vi "PhotonVision_ReadTargetData.vi"() -> ()   [LabVIEW 2019]
uses:
  <vilib>/Rock Robotics/WPI/ThirdParty/PhotonVisionLib/PhotonVisionLib.lvlib
  <vilib>/Rock Robotics/WPI/ThirdParty/JAS_Junk/TrajLib/Trajectory_Library.lvlib
  <vilib>/Rock Robotics/Network Tables/NT Write Number.vi
  <vilib>/Rock Robotics/Network Tables/NT Write Boolean.vi
  <vilib>/Rock Robotics/Network Tables/NT Write String.vi
  <vilib>/Rock Robotics/Network Tables/NT Write Integer.vi
  <vilib>/Rock Robotics/Network Tables/NT Write Numeric Array.vi
  <vilib>/Analysis/Matrix/NI_Matrix.lvlib
  <vilib>/Analysis/Matrix/Numeric/Conversions/Matrix To Array - RM.vi
  <vilib>/Rock Robotics/Network Tables/NT Read Boolean.vi
  <vilib>/Rock Robotics/Network Tables/NT Read Integer.vi
  <vilib>/Rock Robotics/WPI/ThirdParty/PhotonVisionLib/TypeDef/TargetCornerType.ctl
  <vilib>/Rock Robotics/WPI/ThirdParty/JAS_Junk/TrajLib/TypeDef/TRANSLATION3D.ctl
  <vilib>/Rock Robotics/WPI/ThirdParty/JAS_Junk/TrajLib/TypeDef/QUATERNION.ctl
  <vilib>/Rock Robotics/WPI/ThirdParty/JAS_Junk/TrajLib/TypeDef/ROTATION3D.ctl
  <vilib>/Rock Robotics/WPI/ThirdParty/JAS_Junk/TrajLib/TypeDef/TRANSFORM3D.ctl
  <vilib>/Rock Robotics/WPI/ThirdParty/PhotonVisionLib/TypeDef/PhotonTrackedTargetType.ctl
  <vilib>/Rock Robotics/WPI/ThirdParty/PhotonVisionLib/TypeDef/PhotonPipelineResultType.ctl
  <vilib>/Rock Robotics/WPI/ThirdParty/PhotonVisionLib/TypeDef/PhotonPNPResultType.ctl
  <vilib>/Rock Robotics/WPI/ThirdParty/PhotonVisionLib/TypeDef/PhotonMultiTargetPNPResultType.ctl
  <vilib>/Rock Robotics/WPI/ThirdParty/VisionLEDModeType.ctl
  <vilib>/Analysis/Matrix/Datatypes/RealMatrix.ctl
panel:
  in  "LEDMode Request":T1
  out "PipelineIndexReq":i64
  in  "PipelineIndex\nRequest":i32
  out "OutputSnapCmd":i64
  out "InputSnapCmd":i64
  in  "OutputSnapshot":bool
  in  "Input Snapshot":bool
  out "DriverModeRequest":bool
  in  "DriverMode":bool
  out "Dist Coeffs":T2
  out "CameraMatrix":T2
  out "IsConnected 2":bool
  out "PipelineIndex":i32
  out "DriverMode":bool
  out "Version":string
  out "LEDMode":T1
  out "size(s)":i32
  out "unsigned byte array":u8[](array[numeric])
  out "error out":errorcluster
  out "New Data":bool
  out "IsConnected":bool
  out "Has Targets":bool
  in  "CameraName":string="HD_Pro_Webcam_C920"
  out "CtrlLibDistToBestTarg\nMeters":dbl
  out "Loop Count":i32
  out "SpecificPhotonTrackedTarget":T3={"Yaw"=0.0, "Pitch"=0.0, "Area"=0.0, "Skew"=0.0, "MinAreaRectCorners"=[], "BestCameraToTarget"={"TRANSLATION3D"={"X"=0.0, "Y"=0.0, "Z"=0.0}, "ROTATION3D"={"Q_quaternion"={"R"=1.0, "V"=[0.0, 0.0, 0.0]}}, "XF"=FALSE}, "FiiducialId"=0, "AltCameraToTarget"={"TRANSLATION3D"={"X"=0.0, "Y"=0.0, "Z"=0.0}, "ROTATION3D"={"Q_quaternion"={"R"=0.0, "V"=[0.0, 0.0, 0.0]}}, "XF"=FALSE}, "PoseAmbiguity"=0.0, "DetectedCorners"=[]} {"AltCameraToTarget"."TRANSLATION3D"."Z" format="%14.3f"; "AltCameraToTarget"."TRANSLATION3D"."Y" format="%14.3f"; "AltCameraToTarget"."TRANSLATION3D"."X" format="%14.3f"; "BestCameraToTarget"."TRANSLATION3D"."Z" format="%14.3f"; "BestCameraToTarget"."TRANSLATION3D"."Y" format="%14.3f"; "BestCameraToTarget"."TRANSLATION3D"."X" format="%14.3f"}
  out "PipelineResult":T9={"TargetCount"=0, "Latency_MilliSec"=0.0, "Targets"=[], "TimeStampSec"=0.0, "PhotonMultiTargetPNPResult"={"PhotonPNPResult"={"IsPresent"=FALSE, "bestReprojErr"=0.0, "altReprojErr"=0.0, "ambiguity"=0.0, "Best"={"TRANSLATION3D"={"X"=0.0, "Y"=0.0, "Z"=0.0}, "ROTATION3D"={"Q_quaternion"={"R"=1.0, "V"=[0.0, 0.0, 0.0]}}, "XF"=FALSE}, "Alt"={"TRANSLATION3D"={"X"=0.0, "Y"=0.0, "Z"=0.0}, "ROTATION3D"={"Q_quaternion"={"R"=1.0, "V"=[0.0, 0.0, 0.0]}}, "XF"=FALSE}}, "FiducialIDsUsed"=[]}} {"PhotonMultiTargetPNPResult"."PhotonPNPResult"."Alt"."TRANSLATION3D"."Z" format="%14.3f"; "PhotonMultiTargetPNPResult"."PhotonPNPResult"."Alt"."TRANSLATION3D"."Y" format="%14.3f"; "PhotonMultiTargetPNPResult"."PhotonPNPResult"."Alt"."TRANSLATION3D"."X" format="%14.3f"; "PhotonMultiTargetPNPResult"."PhotonPNPResult"."Best"."TRANSLATION3D"."Z" format="%14.3f"; "PhotonMultiTargetPNPResult"."PhotonPNPResult"."Best"."TRANSLATION3D"."Y" format="%14.3f"; "PhotonMultiTargetPNPResult"."PhotonPNPResult"."Best"."TRANSLATION3D"."X" format="%14.3f"; "Targets"."AltCameraToTarget"."TRANSLATION3D"."Z" format="%14.3f"; "Targets"."AltCameraToTarget"."TRANSLATION3D"."Y" format="%14.3f"; "Targets"."AltCameraToTarget"."TRANSLATION3D"."X" format="%14.3f"; "Targets"."BestCameraToTarget"."TRANSLATION3D"."Z" format="%14.3f"; "Targets"."BestCameraToTarget"."TRANSLATION3D"."Y" format="%14.3f"; "Targets"."BestCameraToTarget"."TRANSLATION3D"."X" format="%14.3f"}
  out "SpecificTargetFound":bool
  out "TagTarget Index":i32
  in  "Fiiducial ID\n(April Tag Number)":i32
  out "BestTargetFound":bool
  out "BestYaw":dbl
  out "DistanceToBestTarget \nMeters":dbl
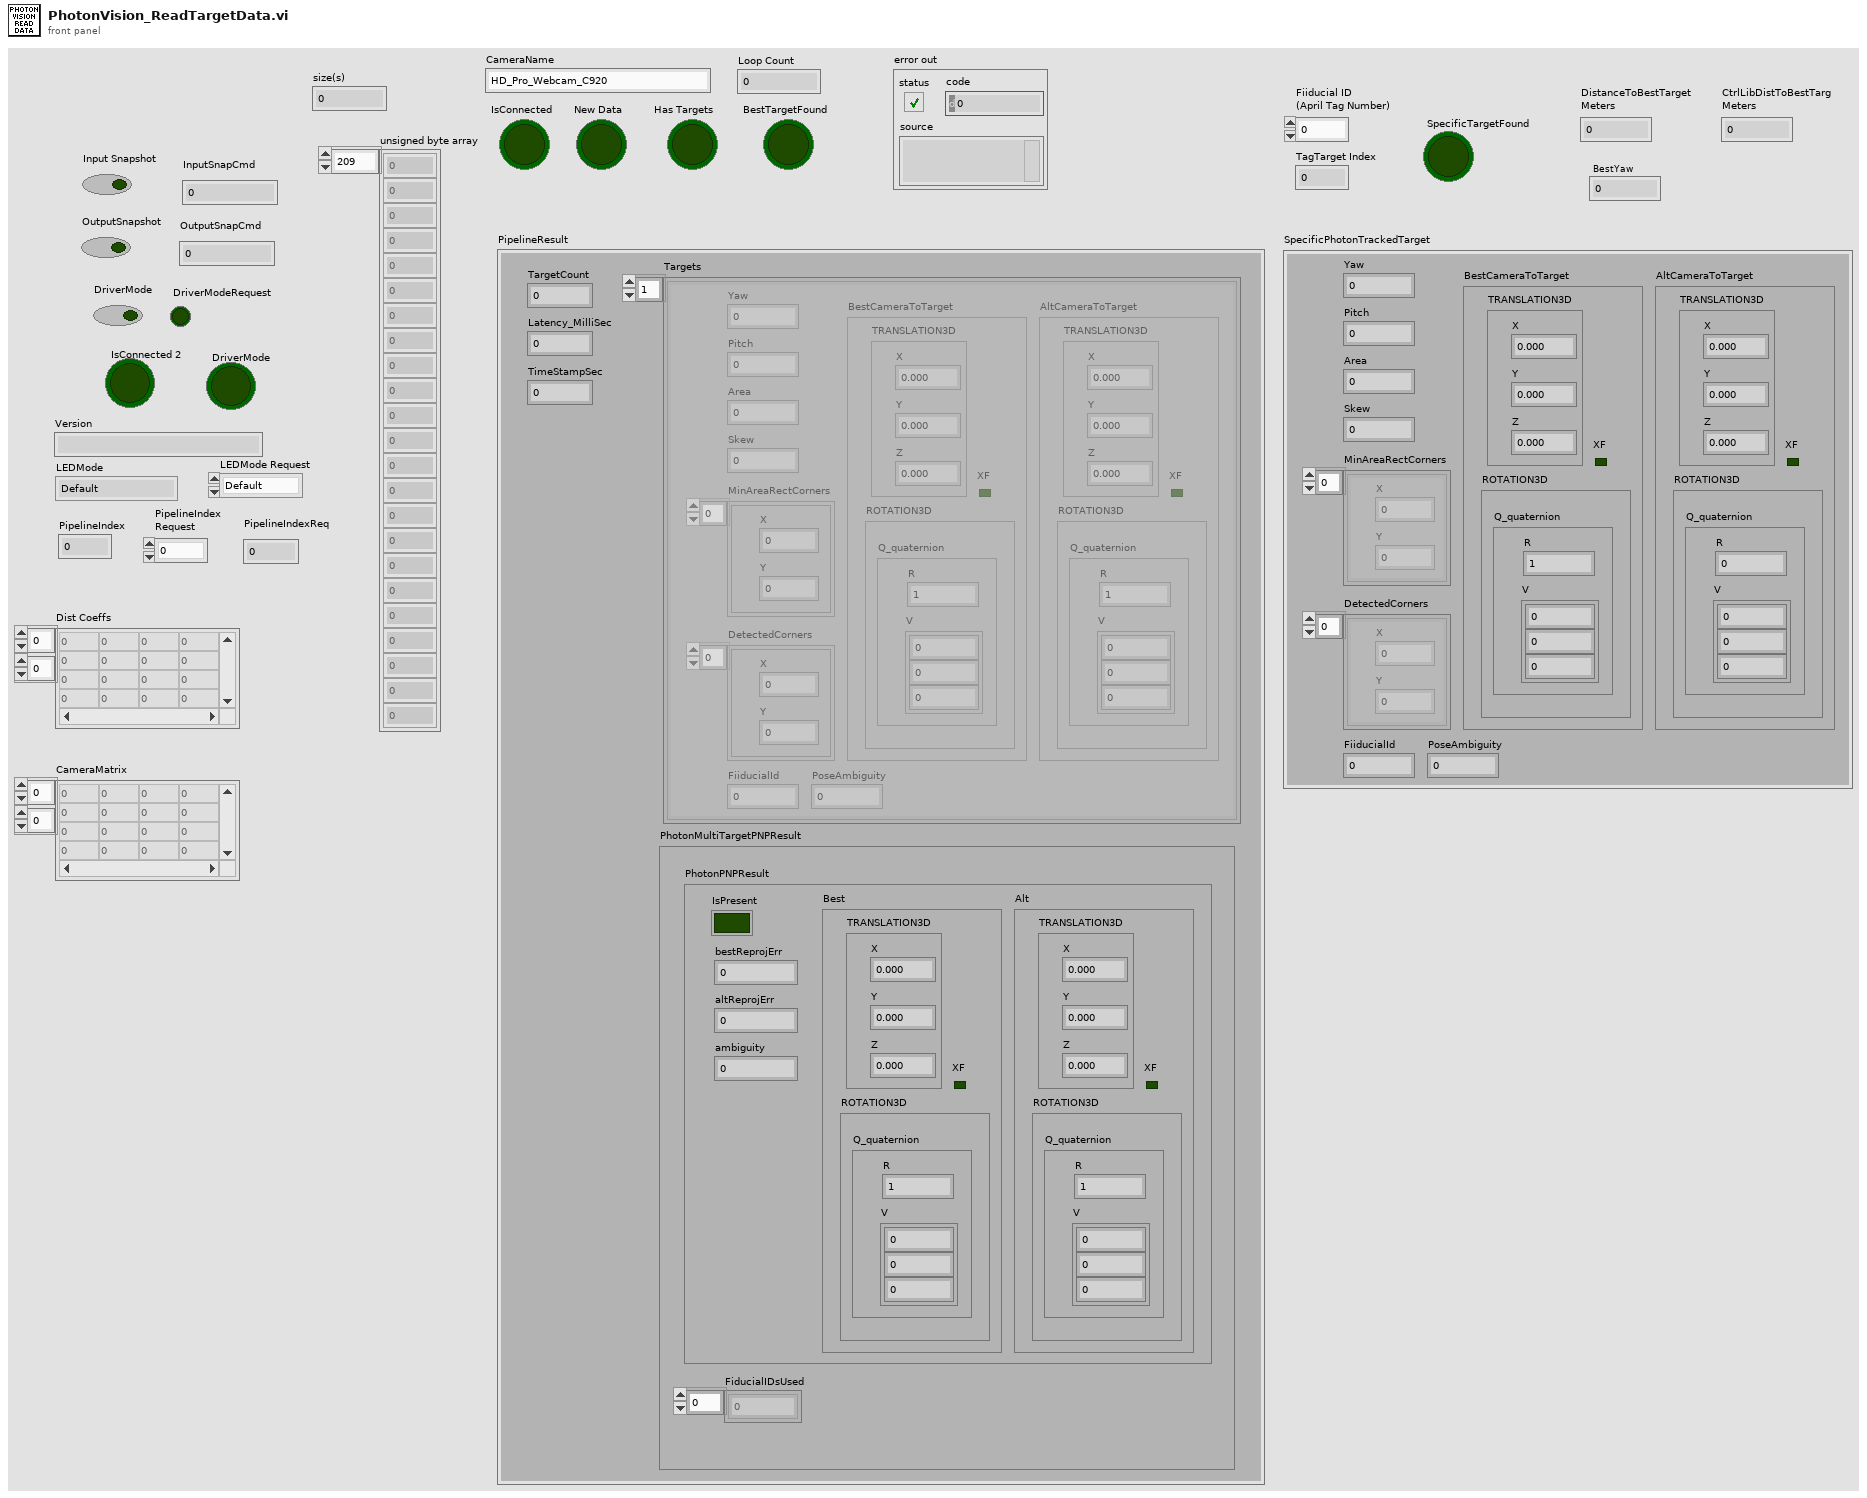
[diagram p1: front panel]
types:
  T1 = typedef "PhotonVisionLib.lvlib/VisionLEDModeType.ctl" = enum16{"Default", "Off", "On", "Blink"}
  T2 = typedef "NI_Matrix.lvlib/RealMatrix.ctl" = dbl[][]
  T3 = typedef "PhotonVisionLib.lvlib/PhotonTrackedTargetType.ctl" = cluster{"Yaw":dbl, "Pitch":dbl, "Area":dbl, "Skew":dbl, "MinAreaRectCorners":T4[], "BestCameraToTarget":T5, "FiiducialId":i32, "AltCameraToTarget":T5, "PoseAmbiguity":dbl, "DetectedCorners":T4[]}
  T4 = typedef "PhotonVisionLib.lvlib/TargetCornerType.ctl" = cluster{"X":dbl, "Y":dbl}
  T5 = typedef "Trajectory_Library.lvlib/TRANSFORM3D.ctl" = cluster{"TRANSLATION3D":T6, "ROTATION3D":T7, "XF":bool}
  T6 = typedef "Trajectory_Library.lvlib/TRANSLATION3D.ctl" = cluster{"X":dbl, "Y":dbl, "Z":dbl}
  T7 = typedef "Trajectory_Library.lvlib/ROTATION3D.ctl" = cluster{"Q_quaternion":T8}
  T8 = typedef "Trajectory_Library.lvlib/QUATERNION.ctl" = cluster{"R":dbl, "V":dbl[]}
  T9 = typedef "PhotonVisionLib.lvlib/PhotonPipelineResultType.ctl" = cluster{"TargetCount":i32, "Latency_MilliSec":dbl, "Targets":T3[], "TimeStampSec":dbl, "PhotonMultiTargetPNPResult":T10}
  T10 = typedef "PhotonVisionLib.lvlib/PhotonMultiTargetPNPResultType.ctl" = cluster{"PhotonPNPResult":T11, "FiducialIDsUsed":i16[]}
  T11 = typedef "PhotonVisionLib.lvlib/PhotonPNPResultType.ctl" = cluster{"IsPresent":bool, "bestReprojErr":dbl, "altReprojErr":dbl, "ambiguity":dbl, "Best":T5, "Alt":T5}
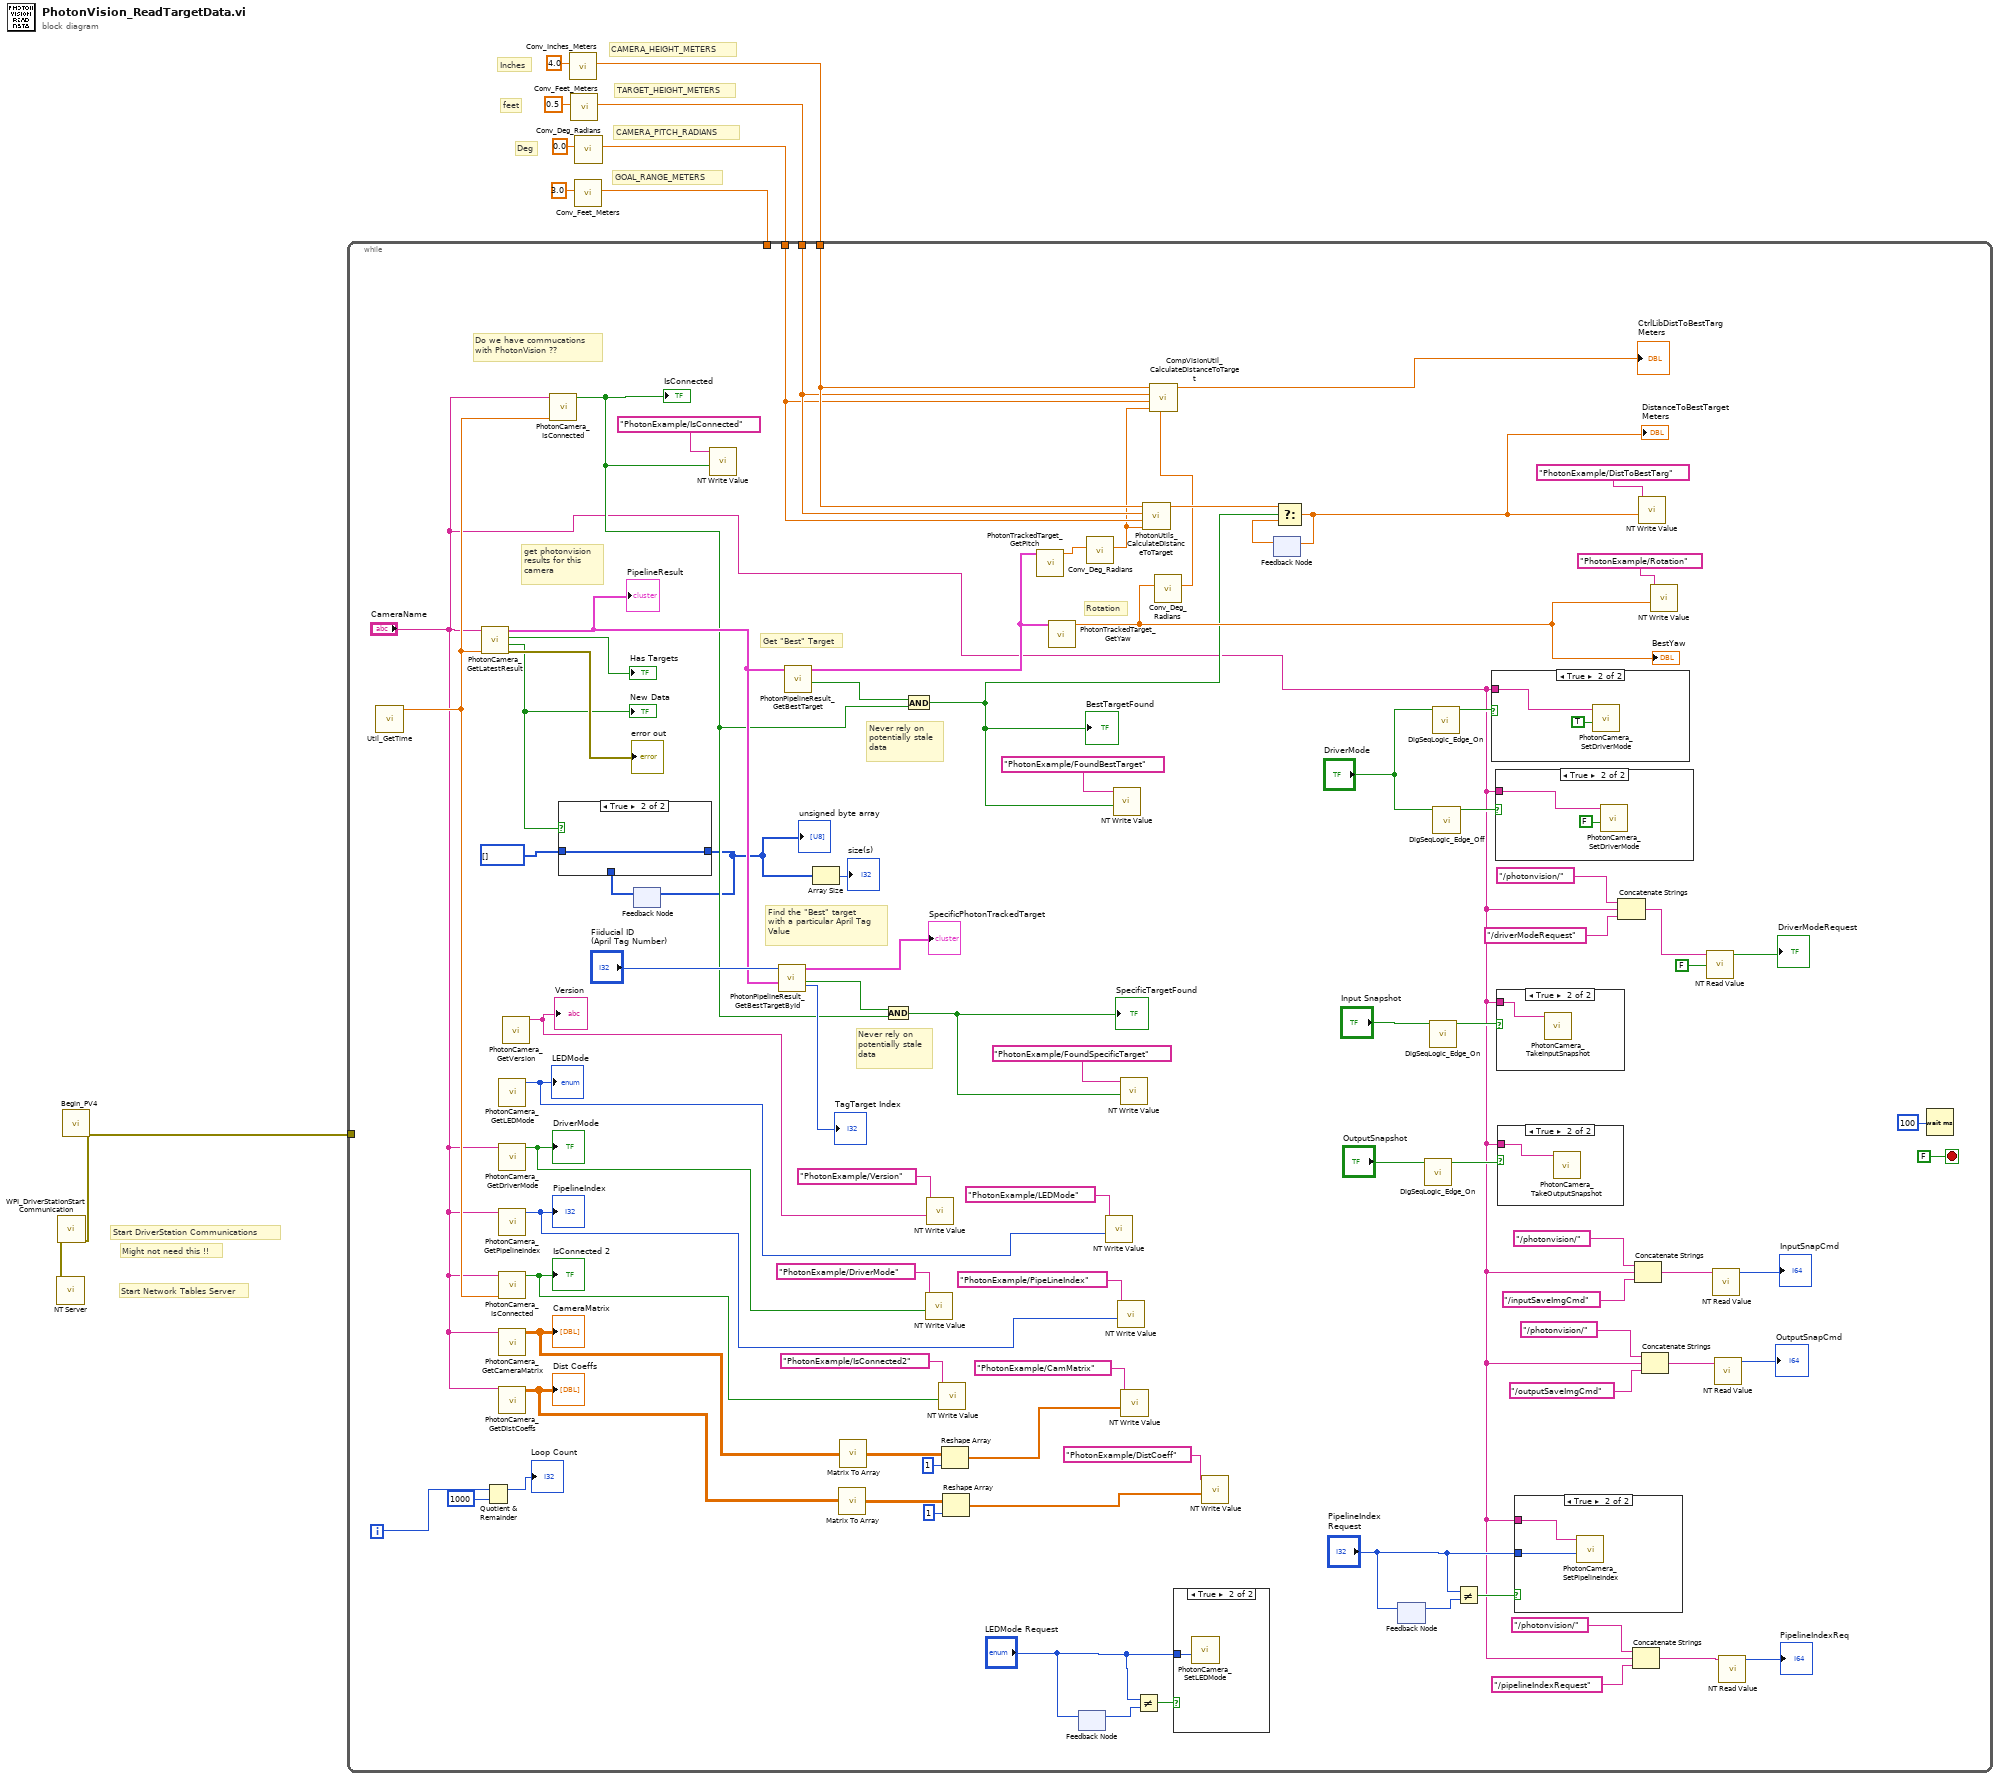
[diagram p0: block diagram]
diagram:
  # "Might not need this !!"
  # "Deg"
  # "feet"
  # "Inches"
  # "GOAL_RANGE_METERS"
  # "CAMERA_PITCH_RADIANS"
  # "TARGET_HEIGHT_METERS"
  # "CAMERA_HEIGHT_METERS"
  # "Start Network Tables Server"
  # "Start DriverStation Communications"
  n1 = call "Begin_PV4.vi"() -> ("error out"=w1:errorcluster)  [unwired: 11 in]
  n2 = call <vilib>:"NT Server.vi"("error in (no error)"=w1) -> ()  [unwired: 10 in, 1 out]
  n3 = call <vilib>:"WPI_DriverStationStart Communication.vi"("error in (no error)"=w1) -> ()  [unwired: 11 in]
  n4 = call <vilib>:"Conv_Inches_Meters.vi"("INCH"=4.0) -> ("Meters"=w5:dbl)  [unwired: 10 in]
  n5 = call <vilib>:"Conv_Feet_Meters.vi"("Feet"=0.5) -> ("Meters"=w4:dbl)  [unwired: 10 in]
  n6 = call <vilib>:"Conv_Feet_Meters.vi"("Feet"=3.0) -> ("Meters"=w2:dbl)  [unwired: 10 in]
  n7 = call <vilib>:"Conv_Deg_Radians.vi"("Degress"=0.0) -> ("Radians"=w3:dbl)  [unwired: 10 in]
  n8 = while {
    tunnel: w5 -> [w81]
    tunnel: w4 -> [w80]
    tunnel: w3 -> [w79]
    tunnel: w2 -> [_]
    tunnel: w1 -> [_]
    i -> [w84]
    stop <- FALSE stop-if-true
    # "Never rely on\npotentially stale\ndata"
    # "Never rely on\npotentially stale\ndata"
    # "Do we have commucations\nwith PhotonVision ??"
    # "Find the \"Best\" target\nwith a particular April Tag\nValue"
    # "Get \"Best\" Target"
    # "Rotation"
    # "get photonvision\nresults for this\ncamera"
    n9 = call <vilib>:"Util_GetTime.vi"() -> ("FPGA_Time_Seconds"=w63:dbl)  [unwired: 9 in, 2 out]
    n10 = call <vilib>:"PhotonCamera_GetLatestResult.vi"("Pass_Through_Time"=w63, "CameraName"="CameraName") -> ("error out"=→"error out":errorcluster, "New Data"=w66:bool, "HasTargets"=→"Has Targets":bool, "PipelineResult"=w88:T9)  [unwired: 6 in]
    "PipelineResult" <- w88
    "New Data" <- w66
    n11 = Quotient & Remainder(x=w84, y=1000) -> (x-y*floor(x/y)=→"Loop Count":i32)  [unwired: 1 out]
    n12 = call <vilib>:"PhotonCamera_GetLEDMode.vi"() -> ("LEDMode"=w59:T1)  [unwired: 10 in, 1 out]
    "LEDMode" <- w59
    n13 = call <vilib>:"PhotonCamera_GetDriverMode.vi"("CameraName"="CameraName") -> ("DriverMode"=w57:bool)  [unwired: 9 in, 1 out]
    "DriverMode" <- w57
    n14 = call <vilib>:"PhotonCamera_GetPipelineIndex.vi"("CameraName"="CameraName") -> ("PipelineIndex"=w55:i32)  [unwired: 9 in, 1 out]
    "PipelineIndex" <- w55
    n15 = call <vilib>:"PhotonCamera_IsConnected.vi"("Pass_Through_Time"=w63, "CameraName"="CameraName") -> ("IsConnected"=w53:bool)  [unwired: 8 in, 1 out]
    "IsConnected 2" <- w53
    n16 = call <vilib>:"PhotonCamera_GetCameraMatrix.vi"("CameraName"="CameraName") -> ("CameraMatrix"=w47:T2)  [unwired: 9 in, 1 out]
    "CameraMatrix" <- w47
    n17 = call <vilib>:"PhotonCamera_GetDistCoeffs.vi"("CameraName"="CameraName") -> ("Dist Coeffs"=w46:T2)  [unwired: 9 in, 1 out]
    "Dist Coeffs" <- w46
    n18 = call <vilib>:"PhotonCamera_GetVersion.vi"() -> ("Version"=w61:string)  [unwired: 10 in, 1 out]
    "Version" <- w61
    n19 = call <vilib>:"PhotonCamera_IsConnected.vi"("Pass_Through_Time"=w63, "CameraName"="CameraName") -> ("IsConnected"=w69:bool)  [unwired: 8 in, 1 out]
    "IsConnected" <- w69
    n20 = feedback #1() -> (w64:u8[])  [unwired: 1 in]
    n21 = case shown="True" w66 {
      tunnel: u8[] [] ("unsigned byte array") -> [_ w110]
      tunnel: [w109 w110] -> w33
      tunnel: w64 -> [w109 _]
      frame False {
      }
      frame True {
      }
    }
    "unsigned byte array" <- w33
    n22 = feedback-in #1(w33) -> ()
    n23 = call-poly <vilib>:"NT Write Value.vi"("value"=w69, "name"="PhotonExample/IsConnected" ("Name")) -> ()  [unwired: 9 in, 1 out]
    n24 = call <vilib>:"PhotonPipelineResult_GetBestTargetById.vi"("PhotonPipelineResult"=w88, "FiducialId"="Fiiducial ID\n(April Tag Number)") -> ("Target Found"=w70:bool, "PhotonTrackedTarget"=→"SpecificPhotonTrackedTarget":T3, "Target Index"=→"TagTarget Index":i32)  [unwired: 7 in]
    n25 = call <vilib>:"PhotonPipelineResult_GetBestTarget.vi"("PhotonPipelineResult"=w88) -> ("TargetFound"=w73:bool, "PhotonTrackedTarget"=w89:T3)  [unwired: 9 in]
    n26 = Array Size(array=w33) -> (size(s)=→"size(s)":i32)
    n27 = call-poly <vilib>:"Matrix To Array.vi"("Real Matrix"=w46) -> ("Real 2D Array"=w48:dbl[][])
    n28 = call-poly <vilib>:"Matrix To Array.vi"("Real Matrix"=w47) -> ("Real 2D Array"=w50:dbl[][])
    n29 = And(x=w70, y=w69) -> (x .and. y?=w71:bool)
    "SpecificTargetFound" <- w71
    n30 = And(x=w73, y=w69) -> (x .and. y?=w72:bool)
    "BestTargetFound" <- w72
    n31 = call-poly <vilib>:"NT Write Value.vi"("value"=w57, "name"="PhotonExample/DriverMode") -> ()  [unwired: 9 in, 1 out]
    n32 = call-poly <vilib>:"NT Write Value.vi"("value"=w61, "name"="PhotonExample/Version") -> ()  [unwired: 9 in, 1 out]
    n33 = call-poly <vilib>:"NT Write Value.vi"("value"=w53, "name"="PhotonExample/IsConnected2") -> ()  [unwired: 9 in, 1 out]
    n34 = Reshape Array(w50, 1 ("dimension size")) -> (w45:dbl[])
    n35 = Reshape Array(w48, 1 ("dimension size")) -> (w43:dbl[])
    n36 = call <vilib>:"PhotonTrackedTarget_GetPitch.vi"("TrackedTarget"=w89) -> ("Pitch"=w91:dbl)  [unwired: 10 in]
    n37 = call <vilib>:"PhotonTrackedTarget_GetYaw.vi"("TrackedTarget"=w89) -> ("Yaw"=w77:dbl)  [unwired: 10 in]
    "BestYaw" <- w77
    n38 = feedback #2() -> (w12:T1)  [unwired: 1 in]
    n39 = feedback-in #2("LEDMode Request") -> ()
    n40 = call <vilib>:"Conv_Deg_Radians.vi"("Degress"=w91) -> ("Radians"=w78:dbl)  [unwired: 10 in]
    n41 = call-poly <vilib>:"NT Write Value.vi"("value"=w59, "name"="PhotonExample/LEDMode") -> ()  [unwired: 9 in, 1 out]
    n42 = call-poly <vilib>:"NT Write Value.vi"("value"=w72, "name"="PhotonExample/FoundBestTarget" ("Name")) -> ()  [unwired: 9 in, 1 out]
    n43 = call-poly <vilib>:"NT Write Value.vi"("value"=w55, "name"="PhotonExample/PipeLineIndex") -> ()  [unwired: 9 in, 1 out]
    n44 = call-poly <vilib>:"NT Write Value.vi"("value"=w71, "name"="PhotonExample/FoundSpecificTarget" ("Name")) -> ()  [unwired: 9 in, 1 out]
    n45 = call-poly <vilib>:"NT Write Value.vi"("value"=w45, "name"="PhotonExample/CamMatrix") -> ()  [unwired: 9 in, 1 out]
    n46 = Not Equal?(x="LEDMode Request", y=w12) -> (x != y?=w10:bool)
    n47 = call <vilib>:"PhotonUtils_CalculateDistanceToTarget.vi"("TargetPitch_Radians"=w78, "CameraPitch_Radians"=w79, "TargetHeight_Meters"=w80, "CameraHeight_Meters"=w81) -> ("DistanceToTarget_Meters"=w94:dbl)  [unwired: 7 in]
    n48 = call <vilib>:"Conv_Deg_Radians.vi"("Degress"=w77) -> ("Radians"=w76:dbl)  [unwired: 10 in]
    n49 = call <vilib>:"CompVisionUtil_CalculateDistanceToTarget.vi"("TargetYawRadians"=w76, "targetPitch_Radians"=w78, "cameraPitch_Radians"=w79, "targetHeight_Meters"=w80, "cameraHeight_Meters"=w81) -> ("DistanceToTarget_Meters"=→"CtrlLibDistToBestTarg\nMeters":dbl)  [unwired: 6 in]
    n50 = case shown="True" w10 {
      tunnel: "LEDMode Request" -> [_ w100]
      frame False {
      }
      frame True {
        n51 = call <vilib>:"PhotonCamera_SetLEDMode.vi"("LEDMode"=w100) -> ()  [unwired: 10 in, 1 out]
      }
    }
    n52 = call-poly <vilib>:"NT Write Value.vi"("value"=w43, "name"="PhotonExample/DistCoeff") -> ()  [unwired: 9 in, 1 out]
    n53 = feedback #3() -> (w92:dbl)  [unwired: 1 in]
    n54 = Select(t=w94, s=w72, f=w92) -> (s? t:f=w93:dbl)
    "DistanceToBestTarget \nMeters" <- w93
    n55 = feedback-in #3(w93) -> ()
    n56 = feedback-in #4("PipelineIndex\nRequest") -> ()
    n57 = feedback #4() -> (w18:i32)  [unwired: 1 in]
    n58 = call <vilib>:"DigSeqLogic_Edge_On.vi"("Input"="OutputSnapshot") -> ("On Edge"=w29:bool)  [unwired: 10 in]
    n59 = call <vilib>:"DigSeqLogic_Edge_On.vi"("Input"="Input Snapshot") -> ("On Edge"=w31:bool)  [unwired: 10 in]
    n60 = call <vilib>:"DigSeqLogic_Edge_On.vi"("Input"="DriverMode") -> ("On Edge"=w40:bool)  [unwired: 10 in]
    n61 = call <vilib>:"DigSeqLogic_Edge_Off.vi"("Input"="DriverMode") -> ("Off Edge"=w41:bool)  [unwired: 10 in]
    n62 = Not Equal?(x="PipelineIndex\nRequest", y=w18) -> (x != y?=w20:bool)
    n63 = case shown="True" w40 {
      tunnel: "CameraName" -> [_ w107]
      frame False {
      }
      frame True {
        n64 = call <vilib>:"PhotonCamera_SetDriverMode.vi"("DriverMode"=TRUE, "CameraName"=w107) -> ()  [unwired: 9 in, 1 out]
      }
    }
    n65 = case shown="True" w41 {
      tunnel: "CameraName" -> [_ w105]
      frame False {
      }
      frame True {
        n66 = call <vilib>:"PhotonCamera_SetDriverMode.vi"("DriverMode"=FALSE, "CameraName"=w105) -> ()  [unwired: 9 in, 1 out]
      }
    }
    n67 = case shown="True" w31 {
      tunnel: "CameraName" -> [_ w103]
      frame False {
      }
      frame True {
        n68 = call <vilib>:"PhotonCamera_TakeInputSnapshot.vi"("CameraName"=w103) -> ()  [unwired: 10 in, 1 out]
      }
    }
    n69 = case shown="True" w29 {
      tunnel: "CameraName" -> [_ w104]
      frame False {
      }
      frame True {
        n70 = call <vilib>:"PhotonCamera_TakeOutputSnapshot.vi"("CameraName"=w104) -> ()  [unwired: 10 in, 1 out]
      }
    }
    n71 = case shown="True" w20 {
      tunnel: "CameraName" -> [_ w102]
      tunnel: "PipelineIndex\nRequest" -> [_ w101]
      frame False {
      }
      frame True {
        n72 = call <vilib>:"PhotonCamera_SetPipelineIndex.vi"("PipelineIndex"=w101, "CameraName"=w102) -> ()  [unwired: 9 in, 1 out]
      }
    }
    n73 = Concatenate Strings("/photonvision/", "CameraName", "/driverModeRequest") -> (w36:string)
    n74 = Concatenate Strings("/photonvision/", "CameraName", "/pipelineIndexRequest") -> (w13:string)
    n75 = Concatenate Strings("/photonvision/", "CameraName", "/inputSaveImgCmd") -> (w23:string)
    n76 = call-poly <vilib>:"NT Write Value.vi"("value"=w93, "name"="PhotonExample/DistToBestTarg" ("Name")) -> ()  [unwired: 9 in, 1 out]
    n77 = Concatenate Strings("/photonvision/", "CameraName", "/outputSaveImgCmd") -> (w24:string)
    n78 = call-poly <vilib>:"NT Write Value.vi"("value"=w77, "name"="PhotonExample/Rotation" ("Name")) -> ()  [unwired: 9 in, 1 out]
    n79 = call-poly <vilib>:"NT Read Value.vi"("default value"=FALSE ("Default Value"), "name"=w36) -> ("value"=→"DriverModeRequest":bool)  [unwired: 7 in, 2 out]
    n80 = call-poly <vilib>:"NT Read Value.vi"("name"=w23) -> ("value"=→"InputSnapCmd":i64)  [unwired: 8 in, 2 out]
    n81 = call-poly <vilib>:"NT Read Value.vi"("name"=w24) -> ("value"=→"OutputSnapCmd":i64)  [unwired: 8 in, 2 out]
    n82 = call-poly <vilib>:"NT Read Value.vi"("name"=w13) -> ("value"=→"PipelineIndexReq":i64)  [unwired: 8 in, 2 out]
    n83 = Wait (ms)(milliseconds to wait=u32 100) -> ()  [unwired: 1 out]
  }
